vi "Formular Param Replace.vi"(8 "error in (no error)":errorcluster caption="Error In", 9 "Param In":dbl[](array[numeric]), 10 "Param Name":string[](array[string])=["MVC", "t"], 11 "Formular In":string) -> (0 "error out":errorcluster caption="Error Out", 1 "Param Out":dbl[](array[numeric]), 3 "Value Out":dbl)   [LabVIEW 2020]
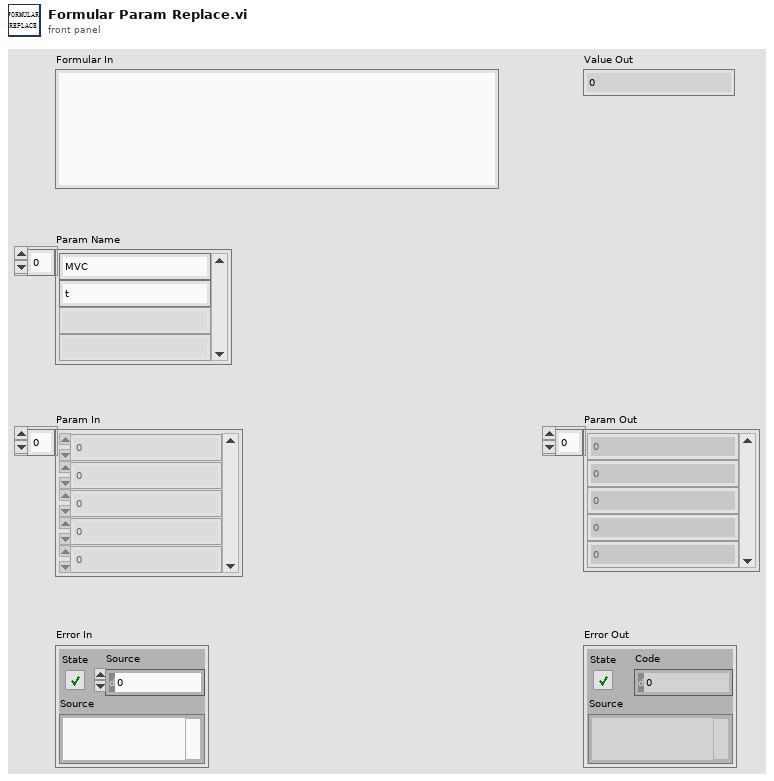
[diagram p1: front panel]
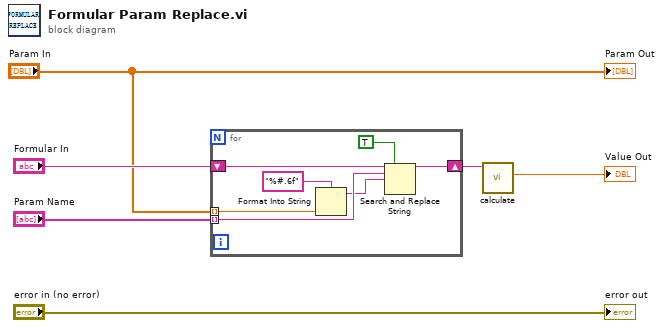
[diagram p0: block diagram]
diagram:
  n1 = for {
    tunnel: "Param Name" -> [w11] mode=indexing
    shift-right: [w8] -> w1
    shift-left: "Formular In" -> [w12]
    tunnel: "Param In" -> [w7] mode=indexing
    n2 = Format Into String(format string="%#.6f" ("格式字符串"), w7) -> (resulting string=w9:string)  [unwired: 2 in, 1 out]
    n3 = Search and Replace String(replace all?=TRUE ("替换全部？(F)"), input string=w12, search string=w11, replace string=w9) -> (result string=w8:string)  [unwired: 4 in, 3 out]
  }
  n4 = call "calculate.vi"("Formular"=w1) -> ("Value"=→"Value Out":dbl)  [unwired: 9 in, 1 out]
  "error out" <- "error in (no error)"
  "Param Out" <- "Param In"
